vi "故障分类表.vi"(8 "低位":i32, 9 "高位":i32, 11 "枚举":T1(ring)) -> (0 "状态":string[](array[string]), 3 "类型":string[](array[string]))   [LabVIEW 2013]
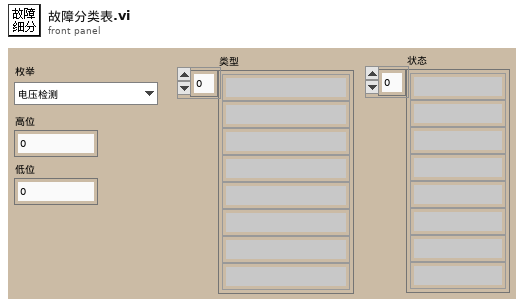
[diagram p1: front panel]
types:
  T1 = enum16{"电压检测", "外总电压检测", "内总电压检测", "温度检测", "电流检测", "绝缘检测", "CAN0检测", "CAN1检测", "CAN4检测", "CAN2检测", "CAN3检测", "RS485检测", "RS232检测", "内部EE存储器", "外部EE存储器", "外部Flash存储器", "CPU", "软件", "DI", "DO", "AI", "AO", "预充电故障", "电池不匹配", "充电异常"}
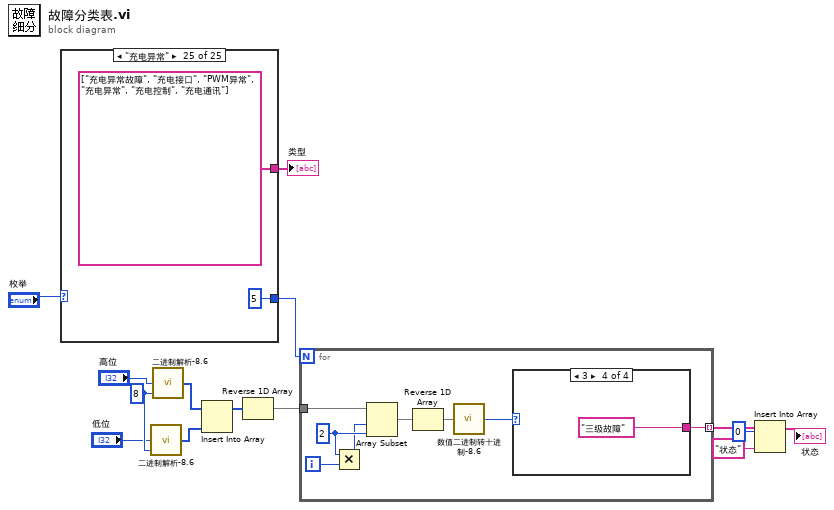
[diagram p0: block diagram]
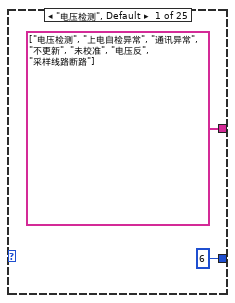
[diagram p2: hidden frame]
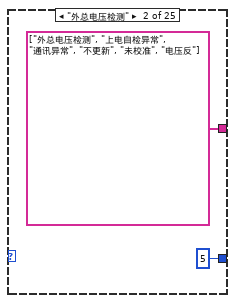
[diagram p3: hidden frame]
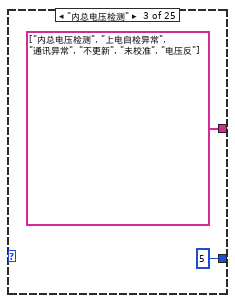
[diagram p4: hidden frame]
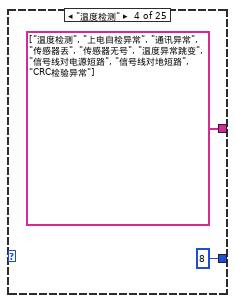
[diagram p5: hidden frame]
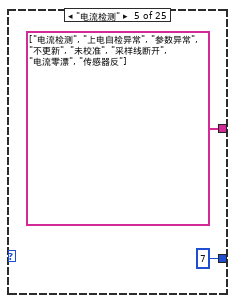
[diagram p6: hidden frame]
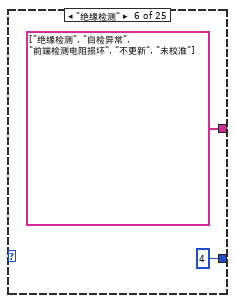
[diagram p7: hidden frame]
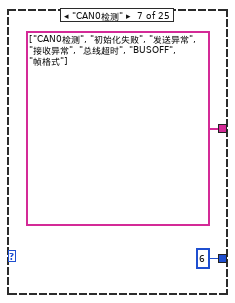
[diagram p8: hidden frame]
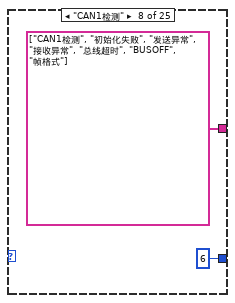
[diagram p9: hidden frame]
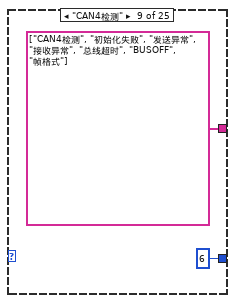
[diagram p10: hidden frame]
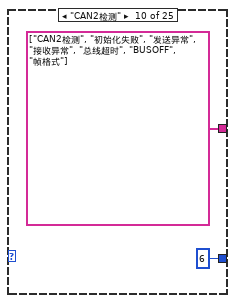
[diagram p11: hidden frame]
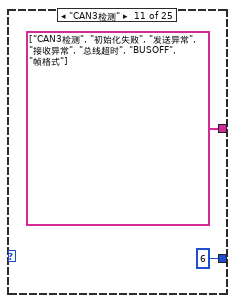
[diagram p12: hidden frame]
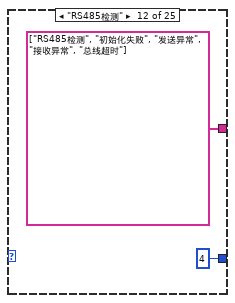
[diagram p13: hidden frame]
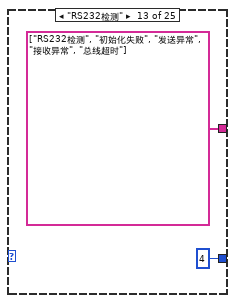
[diagram p14: hidden frame]
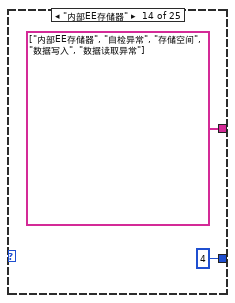
[diagram p15: hidden frame]
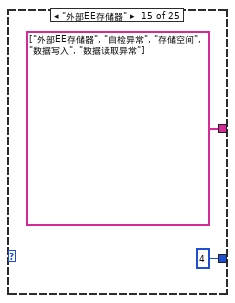
[diagram p16: hidden frame]
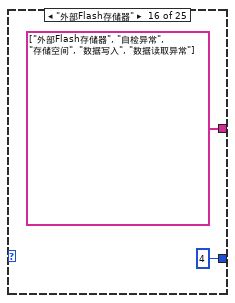
[diagram p17: hidden frame]
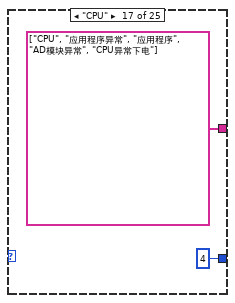
[diagram p18: hidden frame]
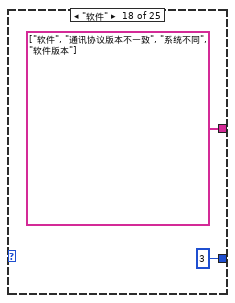
[diagram p19: hidden frame]
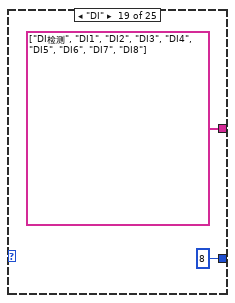
[diagram p20: hidden frame]
diagram:
  w13 = 8 ("索引")
  n1 = case shown="\"充电异常\"" "枚举" {
    tunnel: [6 5 5 8 7 4 6 6 6 6 6 4 4 4 4 4 4 3 8 8 8 8 4 5 5] -> w7
    tunnel: [string[] ["电压检测", "上电自检异常", "通讯异常", "不更新", "未校准", "电压反", "采样线路断路"] string[] ["外总电压检测", "上电自检异常", "通讯异常", "不更新", "未校准", "电压反"] string[] ["内总电压检测", "上电自检异常", "通讯异常", "不更新", "未校准", "电压反"] string[] ["温度检测", "上电自检异常", "通讯异常", "传感器丢", "传感器无号", "温度异常跳变", "信号线对电源短路", "信号线对地短路", "CRC检验异常"] string[] ["电流检测", "上电自检异常", "参数异常", "不更新", "未校准", "采样线断开", "电流零漂", "传感器反"] string[] ["绝缘检测", "自检异常", "前端检测电阻损坏", "不更新", "未校准"] string[] ["CAN0检测", "初始化失败", "发送异常", "接收异常", "总线超时", "BUSOFF", "帧格式"] string[] ["CAN1检测", "初始化失败", "发送异常", "接收异常", "总线超时", "BUSOFF", "帧格式"] string[] ["CAN4检测", "初始化失败", "发送异常", "接收异常", "总线超时", "BUSOFF", "帧格式"] string[] ["CAN2检测", "初始化失败", "发送异常", "接收异常", "总线超时", "BUSOFF", "帧格式"] string[] ["CAN3检测", "初始化失败", "发送异常", "接收异常", "总线超时", "BUSOFF", "帧格式"] string[] ["RS485检测", "初始化失败", "发送异常", "接收异常", "总线超时"] string[] ["RS232检测", "初始化失败", "发送异常", "接收异常", "总线超时"] string[] ["内部EE存储器", "自检异常", "存储空间", "数据写入", "数据读取异常"] string[] ["外部EE存储器", "自检异常", "存储空间", "数据写入", "数据读取异常"] string[] ["外部Flash存储器", "自检异常", "存储空间", "数据写入", "数据读取异常"] string[] ["CPU", "应用程序异常", "应用程序", "AD模块异常", "CPU异常下电"] string[] ["软件", "通讯协议版本不一致", "系统不同", "软件版本"] string[] ["DI检测", "DI1", "DI2", "DI3", "DI4", "DI5", "DI6", "DI7", "DI8"] string[] ["DO检测", "DO1", "DO2", "DO3", "DO4", "DO5", "DO6", "DO7", "DO8"] string[] ["AI检测", "AI1", "AI2", "AI3", "AI4", "AI5", "AI6", "AI7", "AI8"] string[] ["AO检测", "AO1", "AO2", "AO3", "AO4", "AO5", "AO6", "AO7", "AO8"] string[] ["预充电故障", "超时", "后端开路", "后端短路", "预充电回"] string[] ["电池不匹配", "厂家", "电池类型", "SOC状态", "箱间平均", "电池编组"] string[] ["充电异常故障", "充电接口", "PWM异常", "充电异常", "充电控制", "充电通讯"]] -> w2
    frame "电压检测", Default {
    }
    frame "外总电压检测" {
    }
    frame "内总电压检测" {
    }
    frame "温度检测" {
    }
    frame "电流检测" {
    }
    frame "绝缘检测" {
    }
    frame "CAN0检测" {
    }
    frame "CAN1检测" {
    }
    frame "CAN4检测" {
    }
    frame "CAN2检测" {
    }
    frame "CAN3检测" {
    }
    frame "RS485检测" {
    }
    frame "RS232检测" {
    }
    frame "内部EE存储器" {
    }
    frame "外部EE存储器" {
    }
    frame "外部Flash存储器" {
    }
    frame "CPU" {
    }
    frame "软件" {
    }
    frame "DI" {
    }
    frame "DO" {
    }
    frame "AI" {
    }
    frame "AO" {
    }
    frame "预充电故障" {
    }
    frame "电池不匹配" {
    }
    frame "充电异常" {
    }
  }
  "类型" <- w2
  n2 = call "二进制解析-8.6.vi"("索引"=w13, "数值"="低位") -> ("低位子数组"=w10:i32[])  [unwired: 3 out]
  n3 = call "二进制解析-8.6.vi"("索引"=w13, "数值"="高位") -> ("低位子数组"=w11:i32[])  [unwired: 3 out]
  n4 = Insert Into Array(array=w11, new element=w10) -> (w9:i32[])  [unwired: 1 in]
  n5 = Reverse 1D Array(array=w9) -> (reversed array=w8:i32[])
  n6 = for {
    N: w7 -> [_]
    tunnel: w8 -> [w72]
    tunnel: [w65] -> w6 mode=indexing
    i -> [w70]
    w71 = 2
    n7 = Multiply(x=w71, y=w70) -> (x*y=w69:i32)
    n8 = Array Subset(array=w72, index=w69, length=w71) -> (w67:i32[])
    n9 = Reverse 1D Array(array=w67) -> (reversed array=w68:i32[])
    n10 = call "数值二进制转十进制-8.6.vi"("子数组"=w68) -> ("十进制数值"=w66:i32)  [unwired: 4 out]
    n11 = case shown="3" w66 {
      tunnel: ["无故障" "一级故障" "二级故障" "三级故障"] -> w65
      frame 0, Default {
      }
      frame 1 {
      }
      frame 2 {
      }
      frame 3 {
      }
    }
  }
  n12 = Insert Into Array(array=w6, index=0 ("索引"), new element="状态" ("新元素/子数组")) -> (→"状态":string[])
